vi "RSZVB Calibration Standards Catalog With Label.vi"(8 "error in (no error)":errorcluster {"code" format="%.0x"}, 9 "Calibration Kit Label (\"\")":string, 10 "Calibration Kit Name (\"\")":string, 11 "VISA session":refnum<visa-resource-name>) -> (0 "error out":errorcluster {"code" format="%.0x"}, 2 "Catalog":string, 3 "dup VISA session":refnum<visa-resource-name>)   [LabVIEW 2011]
doc: "This VI returns a list of all standards in a given calibration kit.\n\nRemote-control command(s):\n[SENSe<Ch>:]CORRection:CKIT:STANdard:LCATalog? '<ckit_name>', '<ckit_label>'"
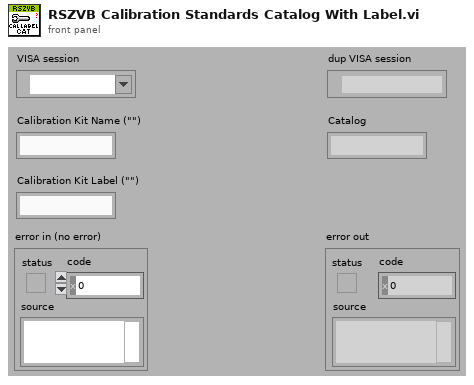
[diagram p1: front panel]
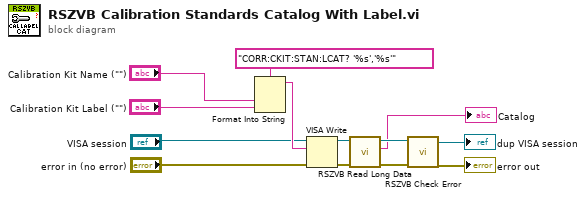
[diagram p0: block diagram]
diagram:
  n1 = Format Into String(format string="CORR:CKIT:STAN:LCAT? '%s','%s'", "Calibration Kit Name (\"\")", "Calibration Kit Label (\"\")") -> (resulting string=w12:string)  [unwired: 2 in, 1 out]
  n2 = VISA Write(VISA resource name="VISA session", write buffer=w12, error in (no error)="error in (no error)") -> (VISA resource name out=w8:refnum<visa-resource-name>, error out=w9:errorcluster)  [unwired: 1 out]
  n3 = call "RSZVB Read Long Data.vi"("error in (no error)"=w9, "VISA resource name"=w8) -> ("error out"=w10:errorcluster, "Data"=→"Catalog":string, "VISA resource name out"=w11:refnum<visa-resource-name>)  [unwired: 7 in]
  n4 = call "RSZVB Check Error.vi"("error in (no error)"=w10, "VISA session"=w11) -> ("error out"=→"error out":errorcluster, "dup VISA session"=→"dup VISA session":refnum<visa-resource-name>)  [unwired: 8 in]
